vi "Find API VI.vi"(8 "error in":errorcluster, 9 "Framework VI to Find":T1, 10 "Library":refnum<class "Library.lvclass">, 11 "Project":refnum<class "Project.lvclass">) -> (0 "error out":errorcluster)   [LabVIEW 2019, in "Panther Dashboard.lvlib"]
uses:
  Panther Dashboard.lvlib
  Public VIs names--enum.ctl
  Class/Library/Library.lvclass
  Class/Project/Project.lvclass
  Class/Library/Library.lvclass/Library.ctl
  Class/Project/Project.lvclass/Project.ctl
  Class/Library/Read Library Ref.vi
  Class/Project/Read Target Ref.vi
  Class/Project/Read Main App Inst Ref.vi
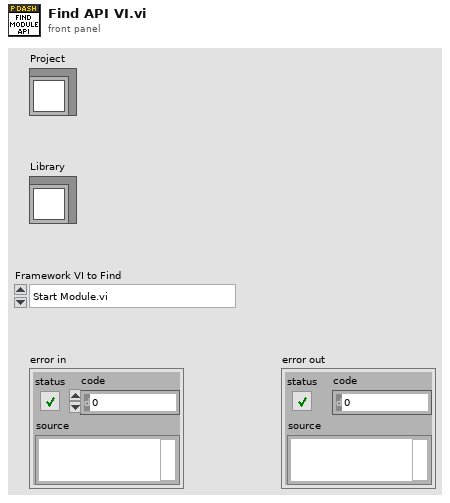
[diagram p1: front panel]
types:
  T1 = typedef "Panther Dashboard.lvlib/Public VIs names--enum.ctl" = enum16{"Start Module.vi", "Synchronize Module Events.vi", "Obtain Broadcast Events for Registration.vi", "Null Broadcast Events--constant.vi", "Stop Module.vi"}
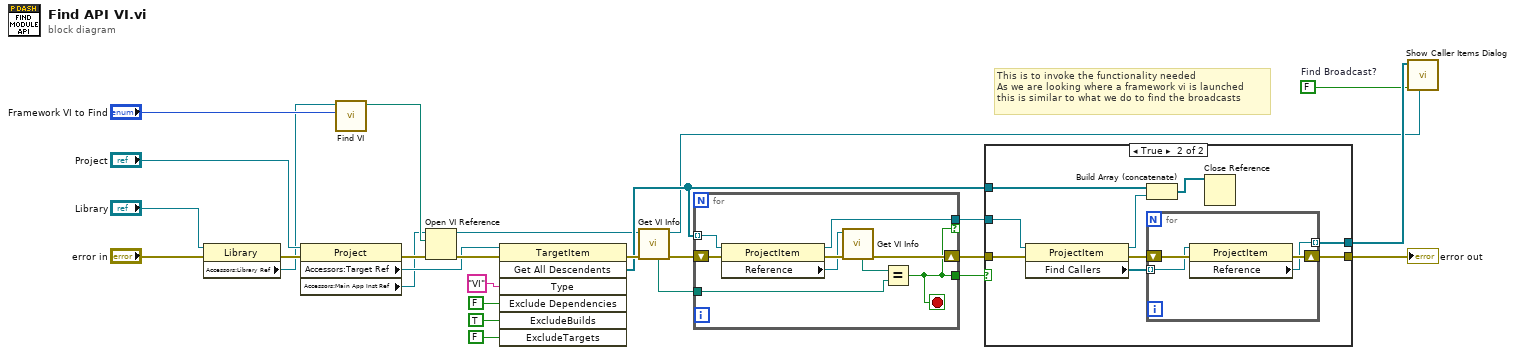
[diagram p0: block diagram]
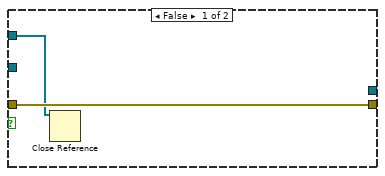
[diagram p2: hidden frame]
diagram:
  w9 = FALSE  # Find Broadcast?
  # "This is to invoke the functionality needed\nAs we are looking where a framework vi is launched\nthis is similar to what we do to find the broadcasts"
  n1 = property class="Library"(reference="Library", error in="error in") -> (error out=w27:errorcluster, "Accessors:Library Ref"=w5:refnum<vi>)  [unwired: 1 out]
  n2 = property class="Project"(reference="Project", error in=w27) -> (error out=w25:errorcluster, "Accessors:Target Ref"=w7:refnum<vi>, "Accessors:Main App Inst Ref"=w4:refnum<vi>)  [unwired: 1 out]
  n3 = call "Find VI.vi"("Framework VI to Find"="Framework VI to Find", "Library in"=w5) -> ("Framework VI Path"=w12:path)  [unwired: 9 in]
  n4 = Open VI Reference(application reference (local)=w4, vi path=w12, error in (no error)=w25) -> (vi reference=w3:refnum<vi>, error out=w24:errorcluster)  [unwired: 3 in]
  n5 = invoke class="TargetItem" method="Get All Descendents"(reference=w7, error in=w24, "Type"="VI", "Exclude Dependencies"=FALSE ("ExcludeDependencies"), "ExcludeBuilds"=TRUE, "ExcludeTargets"=FALSE) -> (error out=w21:errorcluster, "All Descendents"=w13:refnum<vi>[])  [unwired: 1 in, 5 out]
  n6 = call "Get VI Info.vi"("error in"=w21, "VI in"=w3) -> ("error out"=w20:errorcluster, "VI out"=w2:refnum<vi>, "VI Path"=w1:path)  [unwired: 4 in, 3 out]
  n7 = for {
    tunnel: w13 -> [w33] mode=indexing
    tunnel: [w32] -> w17 if=w31
    tunnel: [w31] -> w18
    shift-right: [w34] -> w23
    shift-left: w20 -> [w36]
    tunnel: w1 -> [w30]
    stop <- w31 stop-if-true
    n8 = property class="ProjectItem"(reference=w33, error in=w36) -> (reference out=w32:refnum<vi>, error out=w35:errorcluster, "Reference"=w29:refnum<vi>)
    n9 = call "Get VI Info.vi"("error in"=w35, "VI in"=w29) -> ("error out"=w34:errorcluster, "VI Path"=w28:path)  [unwired: 4 in, 4 out]
    n10 = Equal?(x=w28, y=w30) -> (x = y?=w31:bool)
  }
  n11 = case shown="True" w18 {
    tunnel: w17 -> [_ w44]
    tunnel: w13 -> [w37 w41]
    tunnel: [_ w42] -> w10
    tunnel: w23 -> [w38 w47]
    tunnel: [w38 w45] -> w22
    frame False {
      n12 = Close Reference(reference=w37) -> ()  [unwired: 1 in, 1 out]
    }
    frame True {
      n13 = property class="ProjectItem"(reference=w44, error in=w47) -> (reference out=w39:refnum<vi>, error out=w46:errorcluster, "Find Callers"=w43:refnum<vi>[])
      n14 = Build Array (concatenate)(w41, w39) -> (w40:refnum<vi>[])
      n15 = for {
        tunnel: w43 -> [w49] mode=indexing
        tunnel: [w48] -> w42 mode=indexing
        shift-right: [w50] -> w45
        shift-left: w46 -> [w51]
        n16 = property class="ProjectItem"(reference=w49, error in=w51) -> (error out=w50:errorcluster, "Reference"=w48:refnum<vi>)  [unwired: 1 out]
      }
      n17 = Close Reference(reference=w40) -> ()  [unwired: 1 in, 1 out]
    }
  }
  "error out" <- w22
  n18 = call "Show Caller Items Dialog.vi"("Event"=w2, "Find Broadcast?"=w9, "Request VI Callers"=w10) -> ()  [unwired: 9 in]
